vi "Inject Attribute List.vi"(6 "Attributes Ref":refnum<data-value>, 8 "error in (no error)":errorcluster, 11 "Start Pre-Soak in":refnum<class "Exit.lvclass">) -> (0 "error out":errorcluster, 3 "Start Pre-Soak out":refnum<class "Exit.lvclass">)   [LabVIEW 2019, in "Exit.lvclass"]
uses:
  <vilib>/gpm_packages/@cs/Car-wash/Source/Process Steps/Exit/Exit.lvclass
  <vilib>/gpm_packages/@cs/lookup-table/Source/LookupTable/LookupTable.lvclass
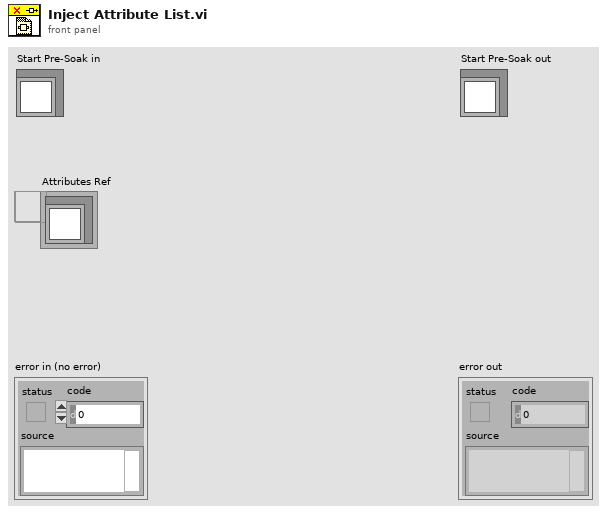
[diagram p1: front panel]
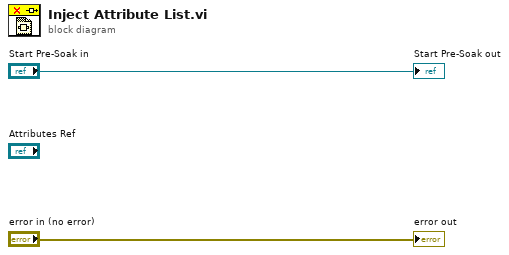
[diagram p0: block diagram]
diagram:
  "error out" <- "error in (no error)"
  "Start Pre-Soak out" <- "Start Pre-Soak in"
